vi "Fit.vi"(7 "Type X":T1(ring), 8 "error in (no error)":errorcluster caption="entrée d'erreur (pas d'erreur)", 9 "y":string[][](array[string]), 10 "X":string[][](array[string]), 11 "QuantileTransformer.lvclass":refnum<class "QuantileTransformer.lvclass">) -> (0 "error out":errorcluster caption="sortie d'erreur", 2 "String Data":string, 3 "QuantileTransformer.lvclass":refnum<class "QuantileTransformer.lvclass">)   [LabVIEW 2020, in "QuantileTransformer.lvclass"]
doc: "Compute the quantiles used for transforming.\n\nReturns : \n\n- String : OK"
uses:
  QuantileTransformer.lvclass
  QuantileTransformer.lvclass/QuantileTransformer.ctl
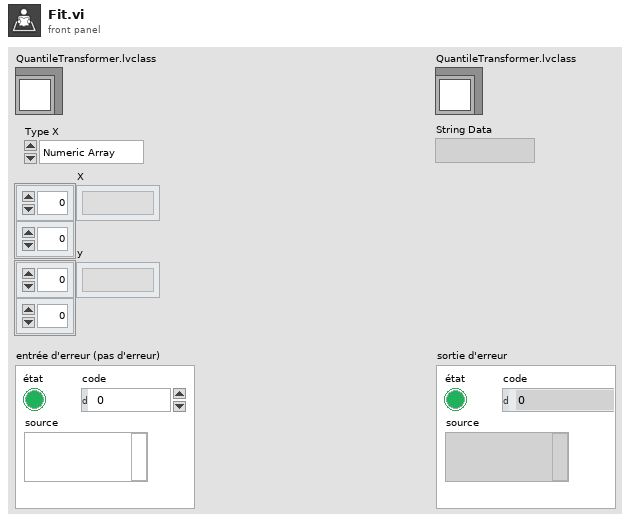
[diagram p1: front panel]
types:
  T1 = enum16{"Numeric Array", "String Array", "Sparse"}
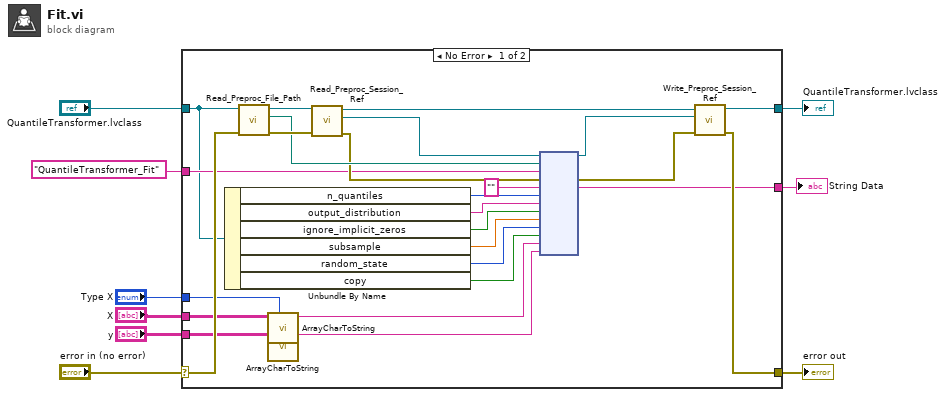
[diagram p0: block diagram]
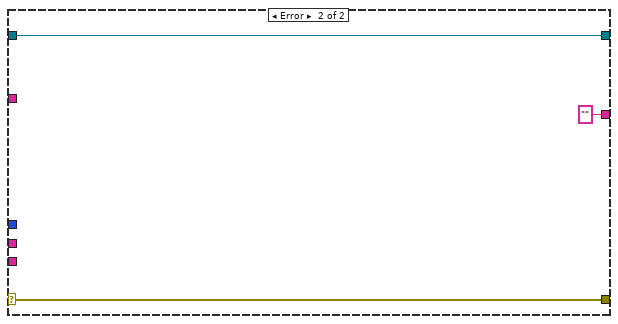
[diagram p2: hidden frame]
diagram:
  n1 = case shown="No Error" "error in (no error)" {
    selector: "error in (no error)" -> [w22 w38]
    tunnel: [w21 w38] -> w8
    tunnel: [w23 w37] -> w6
    tunnel: "QuantileTransformer.lvclass" -> [w18 w37]
    tunnel: "QuantileTransformer_Fit" ("Fonction") -> [w20 _]
    tunnel: [w19 ""] -> w4
    tunnel: "X" -> [w14 _]
    tunnel: "y" -> [w13 _]
    tunnel: "Type X" -> [w12 _]
    frame No Error {
      n2 = Unbundle By Name(w18) -> ("n_quantiles"=w26:i32, "output_distribution"=w25:string, "ignore_implicit_zeros"=w24:bool, "subsample"=w17:dbl, "random_state"=w16:i32, "copy"=w15:bool)
      n3 = call-dynamic "Read_Preproc_File_Path.vi"("error in (no error)"=w22, "Python in"=w18) -> ("error out"=w34:errorcluster, "File_Path"=w31:path, "Python out"=w35:refnum<class "QuantileTransformer.lvclass">)  [unwired: 7 in]
      n4 = call "ArrayCharToString.vi"("Type"=w12, "TAB"=w14) -> ("Instruction"=w11:string)  [unwired: 9 in]
      n5 = call "ArrayCharToString.vi"("TAB"=w13) -> ("Instruction"=w10:string)  [unwired: 10 in]
      n6 = call-dynamic "Read_Preproc_Session_Ref.vi"("error in (no error)"=w34, "Python in"=w35) -> ("error out"=w30:errorcluster, "Session_ref"=w32:refnum<k35>, "Python out"=w33:refnum<class "QuantileTransformer.lvclass">)  [unwired: 7 in]
      n7 = node(w32, w31, w20, w30, "", w26, w25, w24, w17, w16, w15, w11, w10) -> (w28:refnum<k35>, w29:errorcluster, w19:string)  [unwired: 8 in, 2 out]
      n8 = call-dynamic "Write_Preproc_Session_Ref.vi"("error in (no error)"=w29, "Session_ref"=w28, "Python in"=w33) -> ("error out"=w21:errorcluster, "Python out"=w23:refnum<class "QuantileTransformer.lvclass">)  [unwired: 7 in]
    }
    frame Error {
    }
  }
  "error out" <- w8
  "QuantileTransformer.lvclass" <- w6
  "String Data" <- w4
